vi "Cycle and Duration Read Database.vi"(8 "error in (no error)":errorcluster, 10 "Schema":string, 11 "Auto UI in":refnum<class "Auto UI.lvclass">) -> (0 "error out":errorcluster, 2 "Cycles and Duration":T1, 3 "Auto UI out":refnum<class "Auto UI.lvclass">)   [LabVIEW 2023, in "GUI.lvlib" / "Auto UI.lvlib" / "Auto UI.lvclass"]
uses:
  Auto UI.lvclass
  Auto UI.lvclass/Auto UI.ctl
  HardwareAbstractionLayer_LVOOP/Database/Database.lvclass
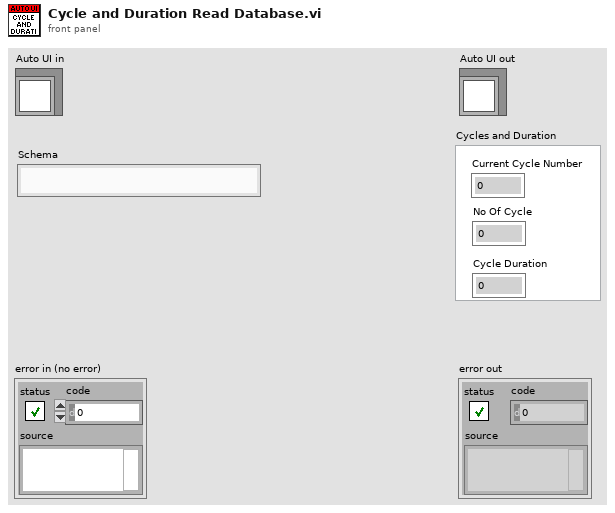
[diagram p1: front panel]
types:
  T1 = cluster{"Current Cycle Number":u32, "No Of Cycle":u32, "Cycle Duration":dbl}
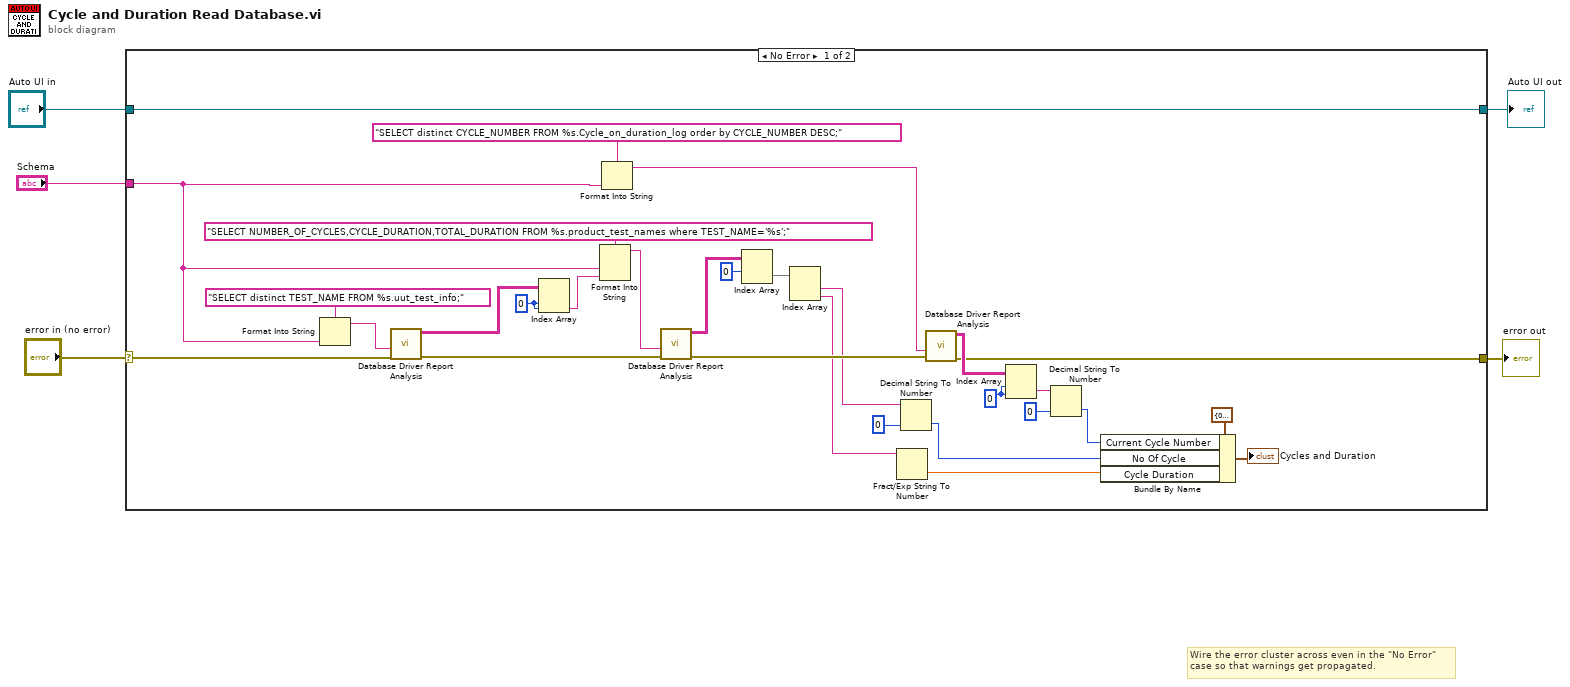
[diagram p0: block diagram]
diagram:
  # "Wire the error cluster across even in the \"No Error\"\ncase so that warnings get propagated."
  n1 = case shown="No Error" "error in (no error)" {
    selector: "error in (no error)" -> [w13 w37]
    tunnel: [w12 w37] -> w4
    tunnel: [w35 w36] -> w2
    tunnel: "Auto UI in" -> [w35 w36]
    tunnel: "Schema" -> [w11 _]
    frame No Error {
      w22 = 0 ("disabled index (col)")
      w31 = 0 ("index (row)")
      n2 = Format Into String(format string="SELECT distinct TEST_NAME FROM %s.uut_test_info;", w11) -> (resulting string=w33:string)  [unwired: 2 in, 1 out]
      n3 = call "Database Driver Report Analysis.vi"("error in"=w13, "SQL query"=w33) -> ("error out"=w29:errorcluster, "data"=w32:string[][])  [unwired: 6 in, 2 out]
      n4 = Index Array(array=w32, index (row)=w31, index (col)=w31) -> (element=w14:string)
      n5 = Format Into String(format string="SELECT NUMBER_OF_CYCLES,CYCLE_DURATION,TOTAL_DURATION FROM %s.product_test_names where TEST_NAME='%s';", w11, w14) -> (resulting string=w28:string)  [unwired: 2 in, 1 out]
      n6 = Format Into String(format string="SELECT distinct CYCLE_NUMBER FROM %s.Cycle_on_duration_log order by CYCLE_NUMBER DESC;", w11) -> (resulting string=w24:string)  [unwired: 2 in, 1 out]
      n7 = call "Database Driver Report Analysis.vi"("error in"=w29, "SQL query"=w28) -> ("error out"=w26:errorcluster, "data"=w27:string[][])  [unwired: 6 in, 2 out]
      n8 = Index Array(array=w27, index (row)=0) -> (element=w18:string[])  [unwired: 1 in]
      n9 = Index Array(array=w18) -> (element #1=w17:string, element #2=w15:string)  [unwired: 2 in]
      n10 = Fract/Exp String To Number(string=w15) -> (number=w7:dbl)  [unwired: 3 in, 1 out]
      n11 = Decimal String To Number(string=w17, default (0L)=u32 0 ("Value")) -> (number=w8:u32)  [unwired: 1 in, 1 out]
      n12 = call "Database Driver Report Analysis.vi"("error in"=w26, "SQL query"=w24) -> ("error out"=w12:errorcluster, "data"=w23:string[][])  [unwired: 6 in, 2 out]
      n13 = Index Array(array=w23, index (row)=w22, index (col)=w22) -> (element=w21:string)
      n14 = Decimal String To Number(string=w21, default (0L)=u32 0 ("Value")) -> (number=w9:u32)  [unwired: 1 in, 1 out]
      n15 = Bundle By Name(cluster=T1 {"Current Cycle Number"=0, "No Of Cycle"=0, "Cycle Duration"=0.0} ("Cycles and Duration"), "Current Cycle Number"=w9, "No Of Cycle"=w8, "Cycle Duration"=w7) -> (→"Cycles and Duration":T1)
    }
    frame Error {
    }
  }
  "error out" <- w4
  "Auto UI out" <- w2
